vi "Video out (SubVI).vi"(11 "ImgData":u8[](array[numeric])) -> (3 "new picture":picture)   [LabVIEW 2014]
uses:
  <vilib>/picture/picture.llb/Draw True-Color Pixmap.vi
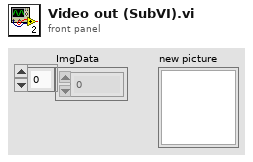
[diagram p1: front panel]
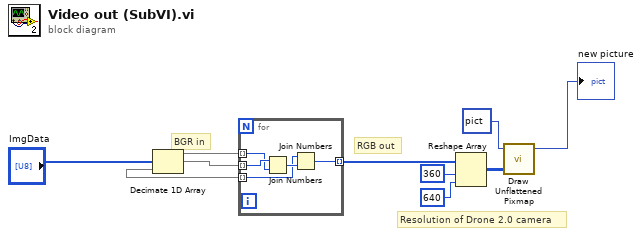
[diagram p0: block diagram]
diagram:
  # "Resolution of Drone 2.0 camera"
  # "RGB out"
  # "BGR in"
  n1 = Decimate 1D Array("ImgData") -> (w6:u8[], w7:u8[], w8:u8[])
  n2 = for {
    tunnel: [w14] -> w1 mode=indexing
    tunnel: w6 -> [w12] mode=indexing
    tunnel: w7 -> [w13] mode=indexing
    tunnel: w8 -> [w11] mode=indexing
    n3 = Join Numbers(hi=w13, lo=w12) -> ((hi.lo)=w15:u16)
    n4 = Join Numbers(hi=w11, lo=w15) -> ((hi.lo)=w14:u32)
  }
  n5 = Reshape Array(w1, 360 ("dimension size"), 640 ("dimension size")) -> (w2:u32[][])
  n6 = call-poly <vilib>:"Draw Unflattened Pixmap.vi"("picture"=picture data[5B], "data (RGB format)"=w2) -> ("new picture"=→"new picture":picture)  [unwired: 7 in]
